vi "用户登录.vi"() -> ()   [LabVIEW 2020]
uses:
  <vilib>/Utility/config.llb/Write Key (String).vi
  <vilib>/Utility/config.llb/NI_LVConfig.lvlib
panel:
  in  "退出":bool
  in  "登录类型：":string(combo)="普通用户"
  in  "密      码：":string
  in  "用      户：":string
  in  "修改密码":bool
  in  "注册":bool
  in  "登录":bool
  out "登录状态":bool
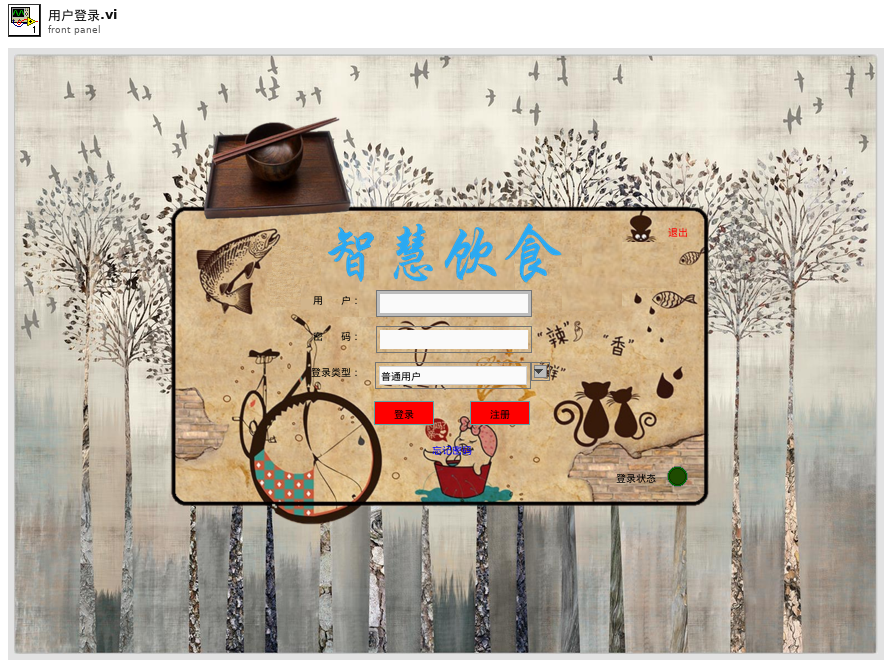
[diagram p1: front panel]
types:
  T1 = enum16{"write", "read", "read_key", "read_section"}
  T2 = enum32{"Invalid", "Standard", "Closed", "Hidden", "Minimized", "Maximized"}
  T3 = typedef "Sound Output Task ID.ctl" = u32
  T4 = typedef "NI_LVConfig.lvlib/Config Data RefNum.ctl" = refnum<k1>
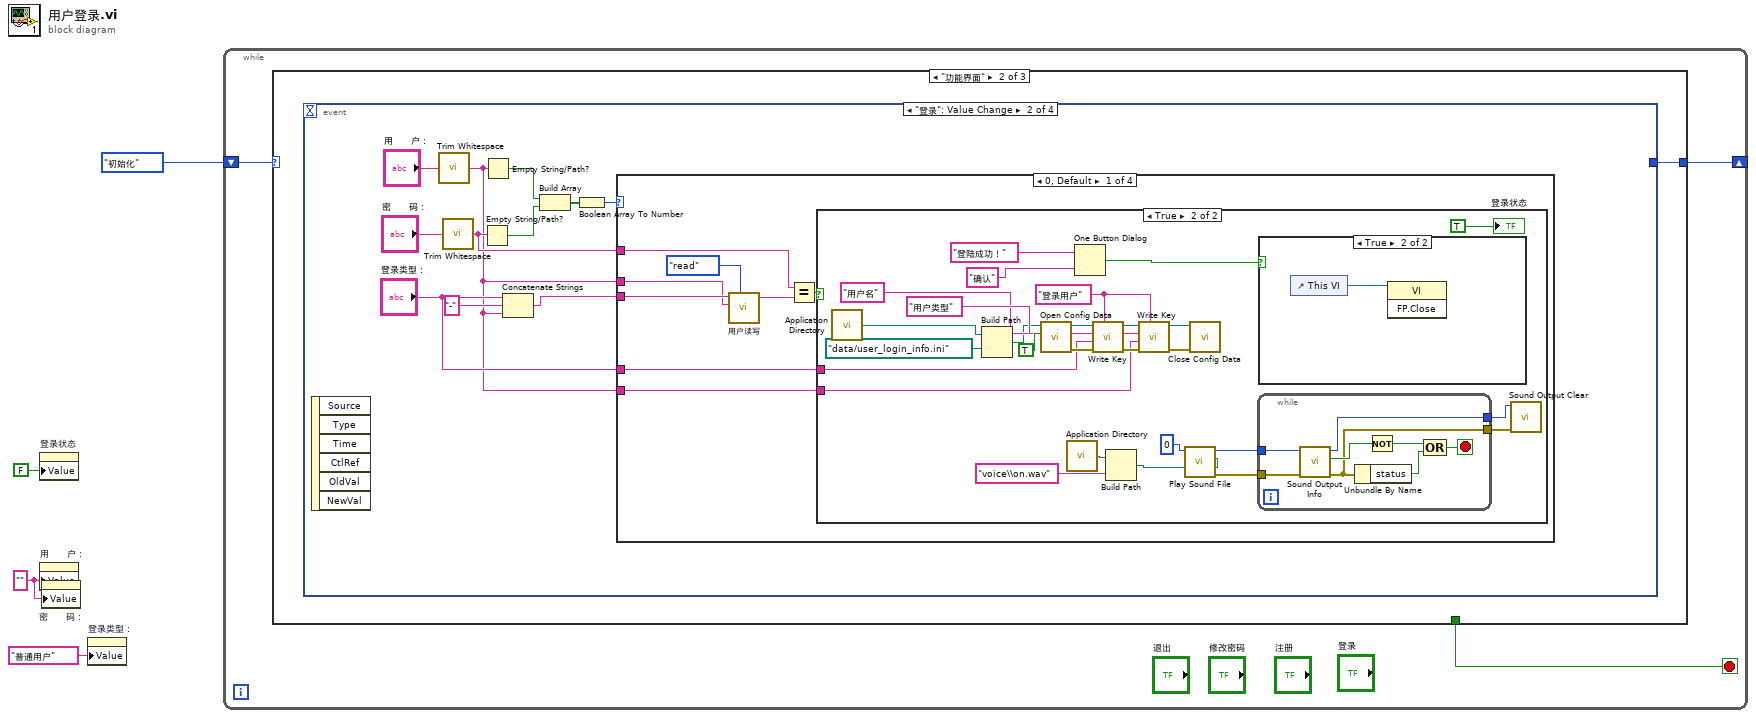
[diagram p0: block diagram]
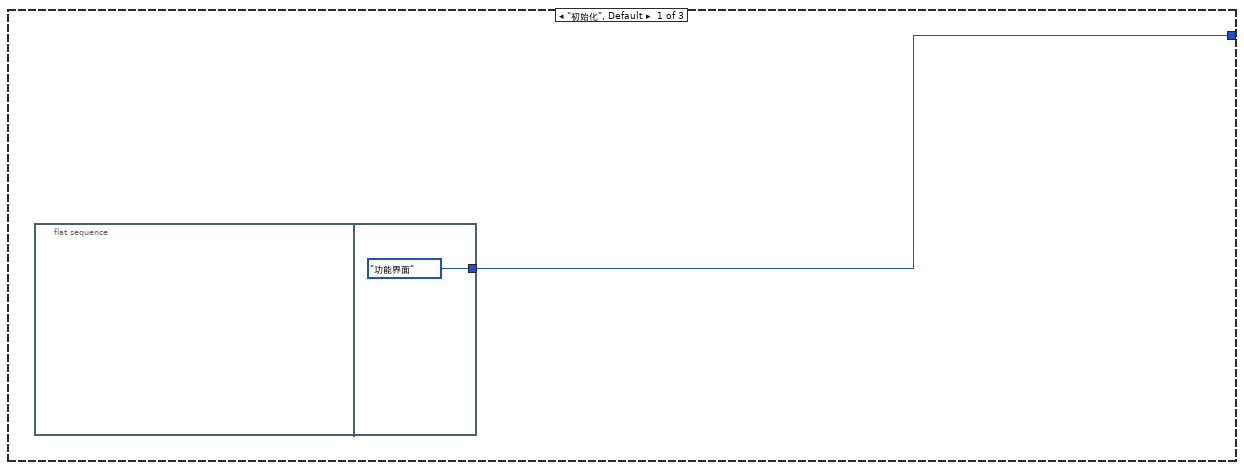
[diagram p2: hidden frame]
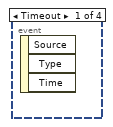
[diagram p3: hidden frame]
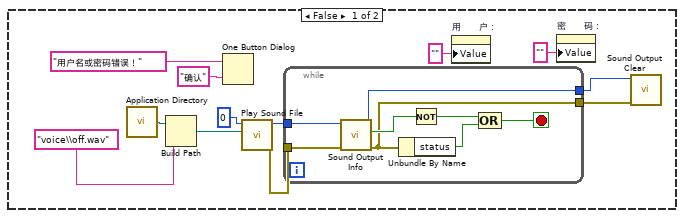
[diagram p4: hidden frame]
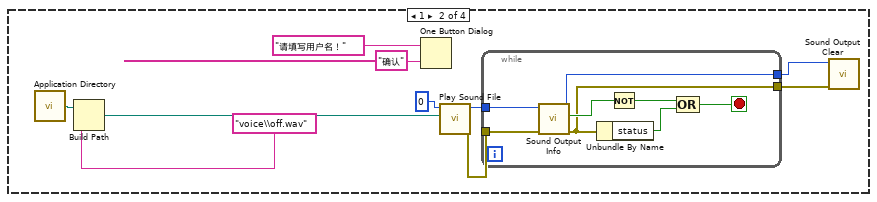
[diagram p6: hidden frame]
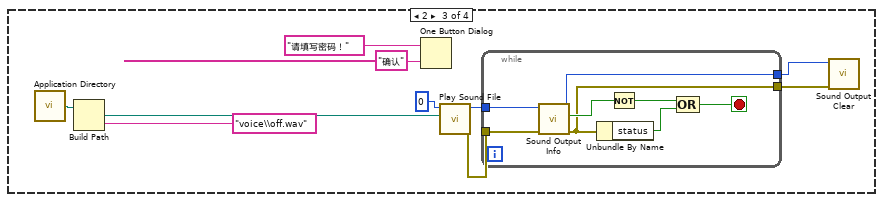
[diagram p7: hidden frame]
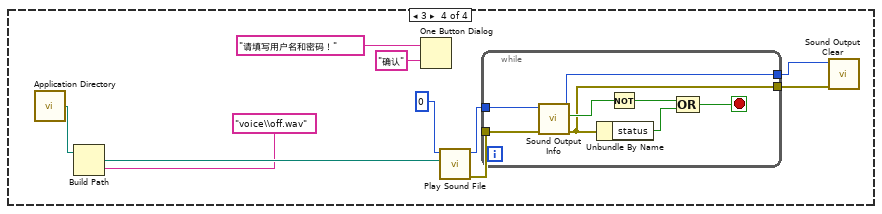
[diagram p8: hidden frame]
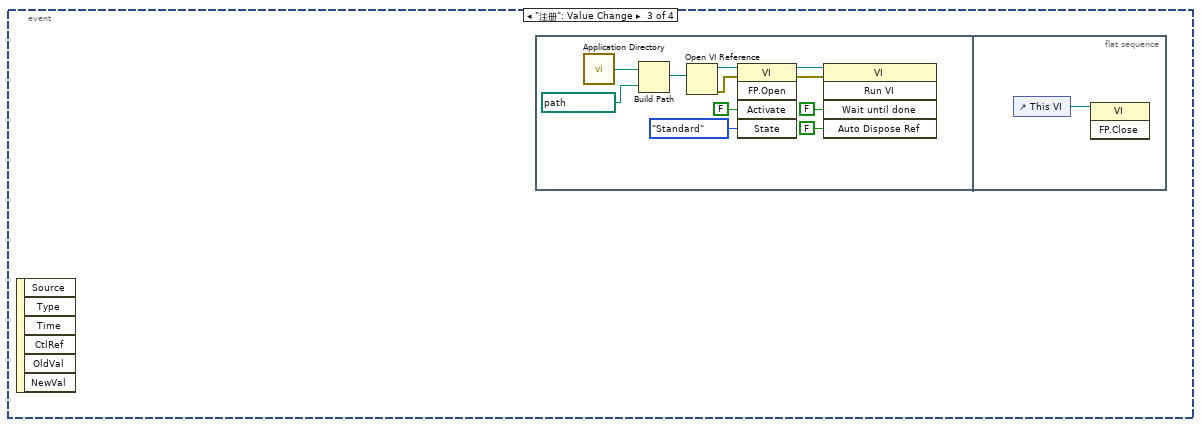
[diagram p9: hidden frame]
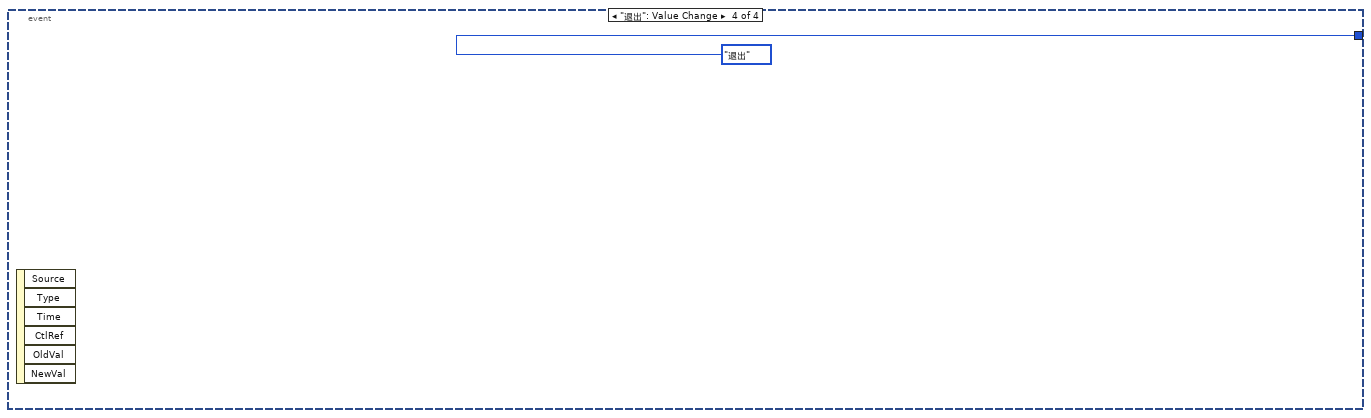
[diagram p10: hidden frame]
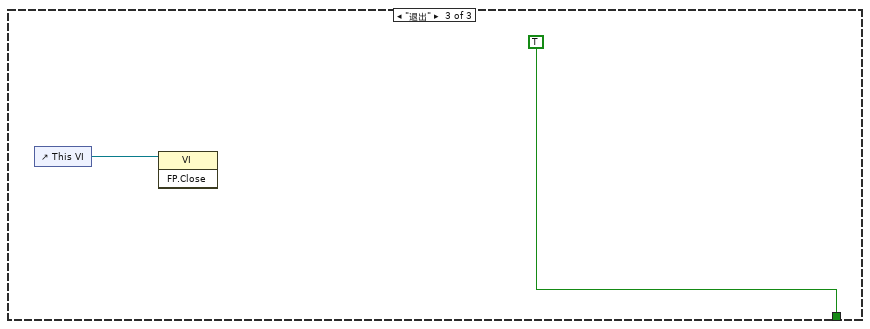
[diagram p11: hidden frame]
diagram:
  w2 = "" ("用户名：")
  n1 = property on="登录状态" class="Bool (strict)"("Value"=FALSE) -> ()  [unwired: 2 in, 2 out]
  n2 = property on="用      户：" class="Str"("Value"=w2) -> ()  [unwired: 2 in, 2 out]
  n3 = property on="密      码：" class="Str"("Value"=w2) -> ()  [unwired: 2 in, 2 out]
  n4 = property on="登录类型：" class="CmbBox"("Value"="普通用户" ("登录类型：")) -> ()  [unwired: 2 in, 2 out]
  n5 = while {
    shift-right: [w6] -> _
    shift-left: enum16{"初始化", "功能界面", "退出"}."初始化" ("功能") -> [w7]
    stop <- w5 stop-if-true
    n6 = case shown="\"功能界面\"" w7 {
      tunnel: [w8 w10 _] -> w6
      tunnel: [_ _ TRUE] -> w5
      frame "初始化", Default {
        n7 = flat-sequence {
          tunnel: [enum16{"初始化", "功能界面", "退出"}."功能界面" ("功能")] -> w8
          frame #0 {
          }
          frame #1 {
          }
        }
      }
      frame "功能界面" {
        n8 = event shown="[1] \"登录\": Value Change" {
          selector: _ -> [_ _ _ _]
          dyn-events: _ -> [_ _ _ _]
          timeout: _ -> [_ _ _ _]
          tunnel: [_ _ _ enum16{"初始化", "功能界面", "退出"}."退出" ("功能")] -> w10
          event Timeout {
            n9 = event-data() -> ()  [unwired: 1 in, 3 out]
          }
          event "登录": Value Change {
            n10 = event-data() -> ()  [unwired: 1 in, 6 out]
            n11 = call <vilib>:"Trim Whitespace.vi"("string"="用      户：") -> ("trimmed string"=w11:string)  [unwired: 1 in]
            n12 = call <vilib>:"Trim Whitespace.vi"("string"="密      码：") -> ("trimmed string"=w13:string)  [unwired: 1 in]
            n13 = Empty String/Path?(string/path=w13) -> (empty?=w18:bool)
            n14 = Empty String/Path?(string/path=w11) -> (empty?=w19:bool)
            n15 = Concatenate Strings("登录类型：", "-" ("string"), w11) -> (w14:string)
            n16 = Build Array(w19, w18) -> (w17:bool[])
            n17 = Boolean Array To Number(Boolean array=w17) -> (number=w16:u32)
            n18 = case shown="0, Default" w16 {
              tunnel: w14 -> [w28 _ _ _]
              tunnel: w11 -> [w27 _ _ _]
              tunnel: w13 -> [w25 _ _ _]
              tunnel: "登录类型：" -> [w23 _ _ _]
              tunnel: w11 -> [w22 _ _ _]
              frame 0, Default {
                n19 = call "用户读写.vi"("Enum"=T1."read", "键"=w27, "字段"=w28) -> ("读取到的值"=w26:string)  [unwired: 6 in, 2 out]
                n20 = Equal?(x=w25, y=w26) -> (x = y?=w24:bool)
                n21 = case shown="True" w24 {
                  tunnel: w23 -> [_ w60]
                  tunnel: w22 -> [_ w56]
                  frame False {
                    n22 = call <vilib>:"Application Directory.vi"() -> ("Application Directory"=w34:path)
                    n23 = Build Path(base path=w34, name or relative path="voice\\off.wav" ("名称或相对路径")) -> (appended path=w39:path)
                    n24 = One Button Dialog(message="用户名或密码错误！" ("消息"), button name ("OK")="确认" ("按钮名称（“确定”）")) -> ()  [unwired: 1 out]
                    n25 = call <vilib>:"Play Sound File.vi"("path"=w39, "device ID"=u32 0) -> ("error out"=w35:errorcluster, "task ID"=w36:T3)  [unwired: 8 in]
                    n26 = while {
                      tunnel: w35 -> [w49]
                      tunnel: w36 -> [w48]
                      tunnel: [w43] -> w37
                      tunnel: [w42] -> w38
                      stop <- w45 stop-if-true
                      n27 = call <vilib>:"Sound Output Info.vi"("error in (no error)"=w49, "task ID"=w48) -> ("error out"=w42:errorcluster, "is playing?"=w47:bool, "task ID out"=w43:T3)  [unwired: 6 in, 1 out]
                      n28 = Unbundle By Name(w42) -> ("status"=w44:bool)
                      n29 = Not(x=w47) -> (.not. x?=w46:bool)
                      n30 = Compound Arithmetic op=OR(w46, w44) -> (w45:bool)
                    }
                    n31 = property on="用      户：" class="Str"("Value"="" ("用      户：")) -> ()  [unwired: 2 in, 2 out]
                    n32 = property on="密      码：" class="Str"("Value"="" ("密      码：")) -> ()  [unwired: 2 in, 2 out]
                    n33 = call <vilib>:"Sound Output Clear.vi"("error in (no error)"=w38, "task ID"=w37) -> ()  [unwired: 9 in, 1 out]
                  }
                  frame True {
                    w58 = "登录用户" ("section")
                    n34 = call <vilib>:"Application Directory.vi"() -> ("Application Directory"=w51:path)
                    n35 = Build Path(base path=w51, name or relative path=path "data/user_login_info.ini") -> (appended path=w50:path)
                    n36 = call <vilib>:"Open Config Data.vi"("create file if necessary (T)"=TRUE, "configuration file path"=w50) -> ("error out"=w63:errorcluster, "refnum"=w62:T4)  [unwired: 7 in, 1 out]
                    n37 = call <vilib>:"Application Directory.vi"() -> ("Application Directory"=w76:path)
                    n38 = One Button Dialog(message="登陆成功！" ("消息"), button name ("OK")="确认" ("按钮名称（“确定”）")) -> (true=w70:bool)
                    n39 = call-poly <vilib>:"Write Key.vi"("section"=w58, "error in (no error)"=w63, "value"=w60, "key"="用户类型", "refnum"=w62) -> ("error out"=w57:errorcluster, "refnum out"=w59:T4)  [unwired: 4 in, 1 out]
                    n40 = Build Path(base path=w76, name or relative path="voice\\on.wav" ("名称或相对路径")) -> (appended path=w71:path)
                    n41 = call-poly <vilib>:"Write Key.vi"("section"=w58, "error in (no error)"=w57, "value"=w56, "key"="用户名", "refnum"=w59) -> ("error out"=w54:errorcluster, "refnum out"=w53:T4)  [unwired: 4 in, 1 out]
                    n42 = call <vilib>:"Play Sound File.vi"("path"=w71, "device ID"=u32 0) -> ("error out"=w75:errorcluster, "task ID"=w74:T3)  [unwired: 8 in]
                    n43 = call <vilib>:"Close Config Data.vi"("error in (no error)"=w54, "refnum"=w53) -> ()  [unwired: 8 in, 2 out]
                    n44 = while {
                      tunnel: w75 -> [w84]
                      tunnel: w74 -> [w83]
                      tunnel: [w78] -> w73
                      tunnel: [w77] -> w72
                      stop <- w80 stop-if-true
                      n45 = call <vilib>:"Sound Output Info.vi"("error in (no error)"=w84, "task ID"=w83) -> ("error out"=w77:errorcluster, "is playing?"=w82:bool, "task ID out"=w78:T3)  [unwired: 6 in, 1 out]
                      n46 = Unbundle By Name(w77) -> ("status"=w79:bool)
                      n47 = Not(x=w82) -> (.not. x?=w81:bool)
                      n48 = Compound Arithmetic op=OR(w81, w79) -> (w80:bool)
                    }
                    n49 = case shown="True" w70 {
                      frame False {
                      }
                      frame True {
                        n50 = control-ref of="This VI"() -> (w85:refnum<vi>)
                        n51 = invoke class="VI" method="FP.Close"(reference=w85) -> ()  [unwired: 2 in, 3 out]
                      }
                    }
                    n52 = call <vilib>:"Sound Output Clear.vi"("error in (no error)"=w72, "task ID"=w73) -> ()  [unwired: 9 in, 1 out]
                    "登录状态" <- TRUE
                  }
                }
              }
              frame 1 {
                n53 = call <vilib>:"Application Directory.vi"() -> ("Application Directory"=w88:path)
                n54 = Build Path(base path=w88, name or relative path="voice\\off.wav" ("名称或相对路径")) -> (appended path=w93:path)
                n55 = One Button Dialog(message="请填写用户名！" ("消息"), button name ("OK")="确认" ("按钮名称（“确定”）")) -> ()  [unwired: 1 out]
                n56 = call <vilib>:"Play Sound File.vi"("path"=w93, "device ID"=u32 0) -> ("error out"=w89:errorcluster, "task ID"=w90:T3)  [unwired: 8 in]
                n57 = while {
                  tunnel: w89 -> [w103]
                  tunnel: w90 -> [w102]
                  tunnel: [w97] -> w91
                  tunnel: [w96] -> w92
                  stop <- w99 stop-if-true
                  n58 = call <vilib>:"Sound Output Info.vi"("error in (no error)"=w103, "task ID"=w102) -> ("error out"=w96:errorcluster, "is playing?"=w101:bool, "task ID out"=w97:T3)  [unwired: 6 in, 1 out]
                  n59 = Unbundle By Name(w96) -> ("status"=w98:bool)
                  n60 = Not(x=w101) -> (.not. x?=w100:bool)
                  n61 = Compound Arithmetic op=OR(w100, w98) -> (w99:bool)
                }
                n62 = call <vilib>:"Sound Output Clear.vi"("error in (no error)"=w92, "task ID"=w91) -> ()  [unwired: 9 in, 1 out]
              }
              frame 2 {
                n63 = call <vilib>:"Application Directory.vi"() -> ("Application Directory"=w106:path)
                n64 = Build Path(base path=w106, name or relative path="voice\\off.wav" ("名称或相对路径")) -> (appended path=w111:path)
                n65 = One Button Dialog(message="请填写密码！" ("消息"), button name ("OK")="确认" ("按钮名称（“确定”）")) -> ()  [unwired: 1 out]
                n66 = call <vilib>:"Play Sound File.vi"("path"=w111, "device ID"=u32 0) -> ("error out"=w107:errorcluster, "task ID"=w108:T3)  [unwired: 8 in]
                n67 = while {
                  tunnel: w107 -> [w121]
                  tunnel: w108 -> [w120]
                  tunnel: [w115] -> w109
                  tunnel: [w114] -> w110
                  stop <- w117 stop-if-true
                  n68 = call <vilib>:"Sound Output Info.vi"("error in (no error)"=w121, "task ID"=w120) -> ("error out"=w114:errorcluster, "is playing?"=w119:bool, "task ID out"=w115:T3)  [unwired: 6 in, 1 out]
                  n69 = Unbundle By Name(w114) -> ("status"=w116:bool)
                  n70 = Not(x=w119) -> (.not. x?=w118:bool)
                  n71 = Compound Arithmetic op=OR(w118, w116) -> (w117:bool)
                }
                n72 = call <vilib>:"Sound Output Clear.vi"("error in (no error)"=w110, "task ID"=w109) -> ()  [unwired: 9 in, 1 out]
              }
              frame 3 {
                n73 = call <vilib>:"Application Directory.vi"() -> ("Application Directory"=w131:path)
                n74 = Build Path(base path=w131, name or relative path="voice\\off.wav" ("名称或相对路径")) -> (appended path=w126:path)
                n75 = One Button Dialog(message="请填写用户名和密码！" ("消息"), button name ("OK")="确认" ("按钮名称（“确定”）")) -> ()  [unwired: 1 out]
                n76 = call <vilib>:"Play Sound File.vi"("path"=w126, "device ID"=u32 0) -> ("error out"=w130:errorcluster, "task ID"=w129:T3)  [unwired: 8 in]
                n77 = while {
                  tunnel: w130 -> [w139]
                  tunnel: w129 -> [w138]
                  tunnel: [w133] -> w128
                  tunnel: [w132] -> w127
                  stop <- w135 stop-if-true
                  n78 = call <vilib>:"Sound Output Info.vi"("error in (no error)"=w139, "task ID"=w138) -> ("error out"=w132:errorcluster, "is playing?"=w137:bool, "task ID out"=w133:T3)  [unwired: 6 in, 1 out]
                  n79 = Unbundle By Name(w132) -> ("status"=w134:bool)
                  n80 = Not(x=w137) -> (.not. x?=w136:bool)
                  n81 = Compound Arithmetic op=OR(w136, w134) -> (w135:bool)
                }
                n82 = call <vilib>:"Sound Output Clear.vi"("error in (no error)"=w127, "task ID"=w128) -> ()  [unwired: 9 in, 1 out]
              }
            }
          }
          event "注册": Value Change {
            n83 = event-data() -> ()  [unwired: 1 in, 6 out]
            n84 = flat-sequence {
              frame #0 {
                n85 = call <vilib>:"Application Directory.vi"() -> ("Application Directory"=w150:path)
                n86 = Build Path(base path=w150, name or relative path=path "用户注册.vi") -> (appended path=w148:path)
                n87 = Open VI Reference(vi path=w148) -> (vi reference=w147:refnum<vi>, error out=w146:errorcluster)  [unwired: 5 in]
                n88 = invoke class="VI" method="FP.Open"(reference=w147, error in=w146, "Activate"=FALSE ("Activate?"), "State"=T2."Standard") -> (reference out=w143:refnum<vi>, error out=w142:errorcluster)  [unwired: 1 in, 3 out]
                n89 = invoke class="VI" method="Run VI"(reference=w143, error in=w142, "Wait until done"=FALSE ("Wait Until Done"), "Auto Dispose Ref"=FALSE ("Auto Dispose Reference")) -> ()  [unwired: 1 in, 5 out]
              }
              frame #1 {
                n90 = control-ref of="This VI"() -> (w151:refnum<vi>)
                n91 = invoke class="VI" method="FP.Close"(reference=w151) -> ()  [unwired: 2 in, 3 out]
              }
            }
          }
          event "退出": Value Change {
            n92 = event-data() -> ()  [unwired: 1 in, 6 out]
          }
        }
      }
      frame "退出" {
        n93 = control-ref of="This VI"() -> (w153:refnum<vi>)
        n94 = invoke class="VI" method="FP.Close"(reference=w153) -> ()  [unwired: 2 in, 3 out]
      }
    }
  }
